vi "Create Data Channel - Array - Type Cast.vi"(8 "error in (no error)":errorcluster, 9 "settings":T2, 10 "channel name":string, 11 "response refnum in":T1 format="%.0x") -> (0 "error out":errorcluster, 1 "channel refnums":T1[](array[typedef]) format="%.0x", 2 "array refnum":T1=18446744073709551615 format="%.0x", 3 "response refnum out":T1 format="%.0x")   [LabVIEW 2020, in "Instrument Addon Scripting API.lvlib"]
doc: "Creates a new Data Channel Array under the specified response."
uses:
  Instrument Addon Scripting API.lvlib
  <vilib>/NI VeriStand/Custom Device API/Custom Device Item Ref.ctl
  TypeDefs/Array Type Cast Settings.ctl
  TypeDefs/Array Element.ctl
  Addon/Addon Shared/Types/Type Cast Type.ctl
  Addon/Addon Shared/Types/Endian.ctl
  Addon/Addon Shared/Types/Data Parameters.ctl
  Addon/Addon Shared/Types/Protocol Data Type.ctl
  Addon/Addon Shared/Types/Data Channel Type.ctl
  Addon/Addon Shared/SubVIs/Constants.vi
  Addon/Addon Shared/Instrument Addon Shared.lvlib
  <vilib>/NI VeriStand/Custom Device API/Custom Device API.lvlib
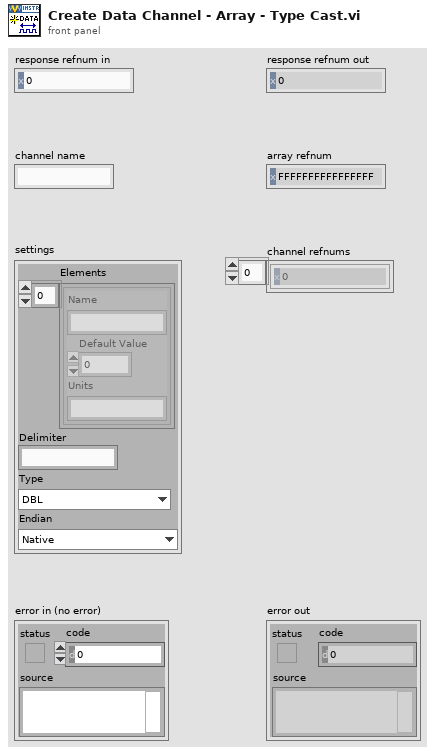
[diagram p1: front panel]
types:
  T1 = typedef "Custom Device API.lvlib/Custom Device Item Ref.ctl" = u64
  T2 = typedef "Instrument Addon Scripting API.lvlib/Array Type Cast Settings.ctl" = cluster{"Elements":T3[], "Delimiter":string, "Type":T4, "Endian":T5}
  T3 = typedef "Instrument Addon Scripting API.lvlib/Array Element.ctl" = cluster{"Name":string, "Default Value":dbl, "Units":string}
  T4 = typedef "Instrument Addon Shared.lvlib/Type Cast Type.ctl" = enum16{"DBL", "SGL", "U64", "U32", "U16", "U8", "I64", "I32", "I16", "I8"}
  T5 = typedef "Instrument Addon Shared.lvlib/Endian.ctl" = enum16{"Native", "Little", "Big"}
  T6 = typedef "Instrument Addon Shared.lvlib/Data Channel Type.ctl" = enum16{"Format", "Comparison", "Type Cast", "Enumerated List"}
  T7 = typedef "Instrument Addon Shared.lvlib/Protocol Data Type.ctl" = enum16{"Single Channel", "Array"}
  T8 = typedef "Instrument Addon Shared.lvlib/Data Parameters.ctl" = cluster{"Data Type":T7, "Channel Type":T6, "Format String":string, "Expected String":string, "Type":T4, "List":string[], "Delimiter":string, "Endian":T5}
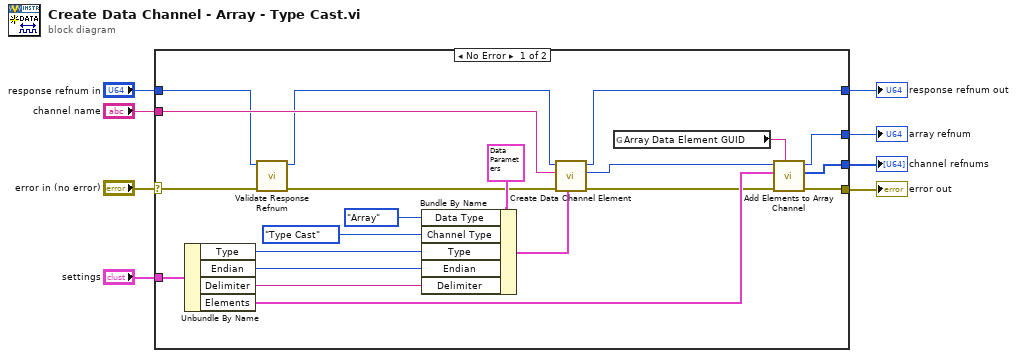
[diagram p0: block diagram]
diagram:
  n1 = case shown="No Error" "error in (no error)" {
    selector: "error in (no error)" -> [w13 w31]
    tunnel: [w24 w31] -> w8
    tunnel: [w15 w30] -> w7
    tunnel: "channel name" -> [w20 _]
    tunnel: "response refnum in" -> [w11 w30]
    tunnel: "settings" -> [w23 _]
    tunnel: [w16 _] -> w2
    tunnel: [w14 _] -> w1
    frame No Error {
      n2 = Unbundle By Name(w23) -> ("Type"=w26:T4, "Endian"=w25:T5, "Delimiter"=w21:string, "Elements"=w22:T3[])
      n3 = call "Validate Response Refnum.vi"("error in (no error)"=w13, "response refnum in"=w11) -> ("error out"=w12:errorcluster, "response refnum out"=w10:T1)  [unwired: 8 in]
      n4 = Bundle By Name(cluster=T8 {"Data Type"=enum."Array", "Channel Type"=enum."Format", "Format String"="%.3g", "Expected String"="", "Type"=enum."SGL", "List"=[], "Delimiter"=",", "Endian"=enum."Native"} ("Settings"), "Data Type"=Protocol_Data_Type."Array", "Channel Type"=Data_Channel_Type."Type Cast", "Type"=w26, "Endian"=w25, "Delimiter"=w21) -> (w19:T8)
      n5 = call "Create Data Channel Element.vi"("Data Channel Parameters"=w19, "Error In"=w12, "Name"=w20, "Refnum In"=w10) -> ("Error Out"=w17:errorcluster, "Channel Refnum"=w18:T1, "Refnum Out"=w15:T1)  [unwired: 5 in]
      n6 = global read "Constants.vi" "Array Data Element GUID"() -> (w9:string)
      n7 = call "Add Elements to Array Channel.vi"("array element GUID"=w9, "error in (no error)"=w17, "array elements"=w22, "array refnum in"=w18) -> ("error out"=w24:errorcluster, "channel refnums"=w16:T1[], "array refnum out"=w14:T1)  [unwired: 5 in]
    }
    frame Error {
    }
  }
  "error out" <- w8
  "response refnum out" <- w7
  "channel refnums" <- w2
  "array refnum" <- w1
